vi "Test Combinations of Broken Wells.vi"(10 "broken streaks":u8[](array[numeric]), 11 "map":i8[](array[numeric])) -> (3 "possible combinations":u64)   [LabVIEW 2022 SP3]
uses:
  <vilib>/Utility/miscctls.llb/LVMapReplaceAction.ctl
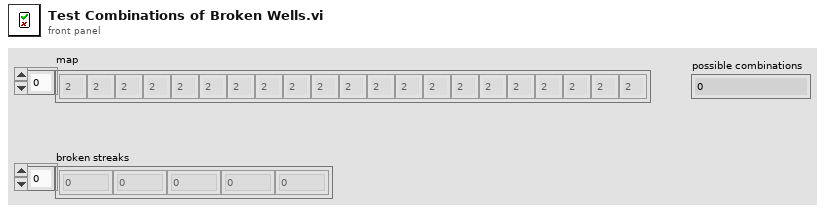
[diagram p1: front panel]
types:
  T1 = typedef "LVMapReplaceAction.ctl" = enum32{"Modify Entry only if found", "Add or Modify Entry", "Delete Entry"}
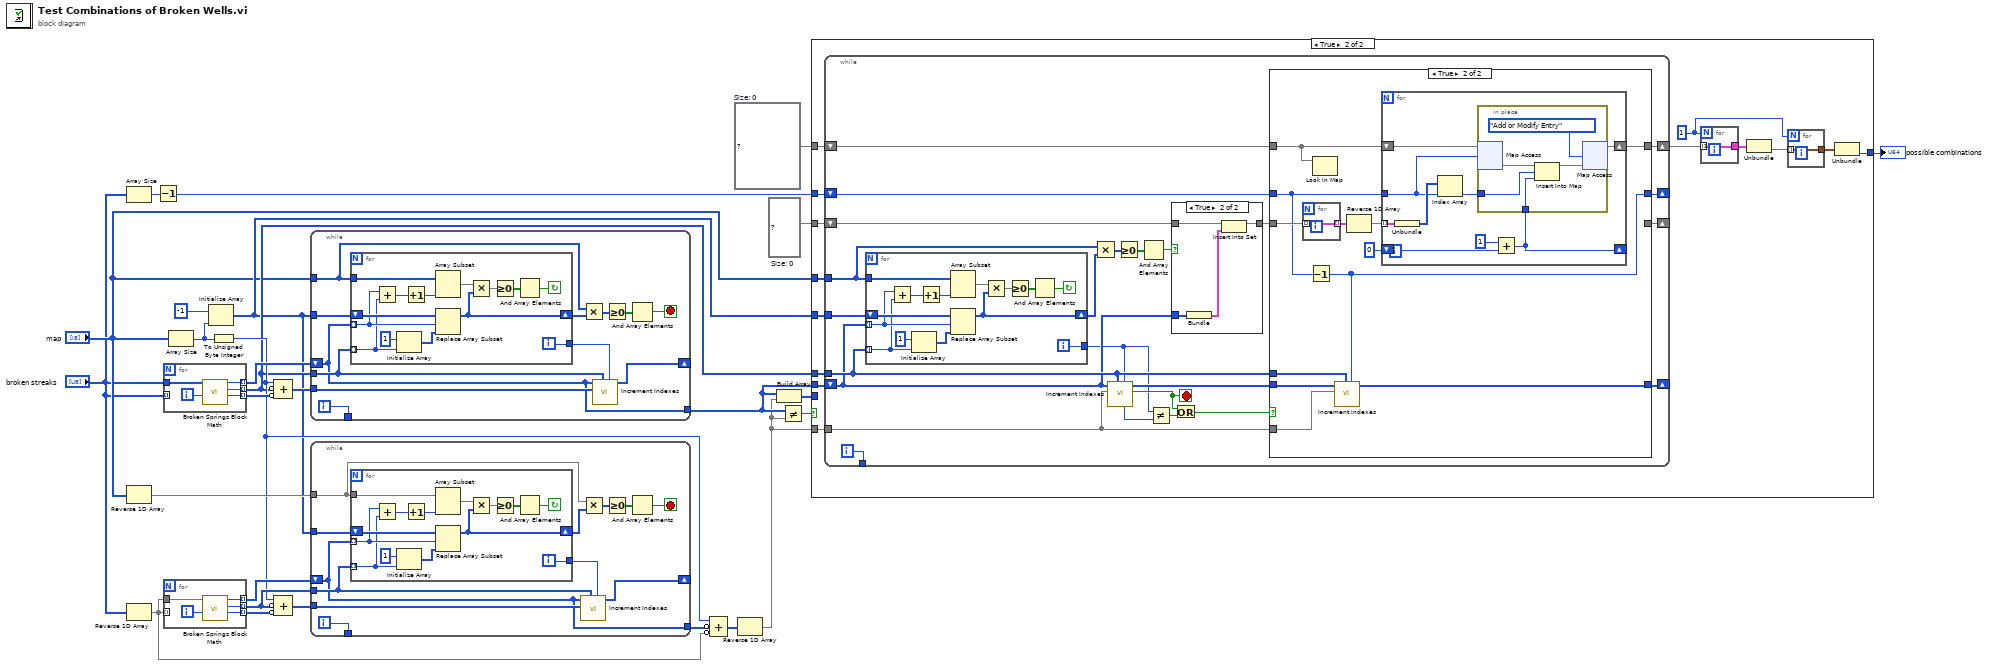
[diagram p0: block diagram]
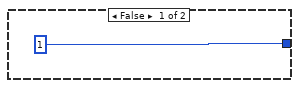
[diagram p2: hidden frame]
diagram:
  w5 = set{cluster{u8[]}} {}  # Size: 0
  w9 = map{i32, map{u8, u64}} {}  # Size: 0
  n1 = Array Size(array="broken streaks") -> (size(s)=w2:i32)
  n2 = Reverse 1D Array(array="map") -> (reversed array=w23:i8[])
  n3 = Reverse 1D Array(array="broken streaks") -> (reversed array=w17:u8[])
  n4 = Decrement(x=w2) -> (x-1=w1:i32)
  n5 = for {
    tunnel: "broken streaks" -> [w32]
    tunnel: "broken streaks" -> [_] mode=indexing
    tunnel: [w30] -> w26 mode=indexing
    tunnel: [w29] -> w11 mode=indexing
    tunnel: [w28] -> w27 mode=indexing
    i -> [w31]
    n6 = call "Broken Springs Block Math.vi"("index"=w31, "contiguous length of broken springs"=w32) -> ("right total"=w28:u8, "current index broken streak length"=w29:u8, "left total"=w30:u8)  [unwired: 7 in]
  }
  n7 = for {
    tunnel: w17 -> [w37]
    tunnel: w17 -> [_] mode=indexing
    tunnel: [w35] -> w21 mode=indexing
    tunnel: [w34] -> w20 mode=indexing
    tunnel: [w33] -> w22 mode=indexing
    i -> [w36]
    n8 = call "Broken Springs Block Math.vi"("index"=w36, "contiguous length of broken springs"=w37) -> ("right total"=w33:u8, "current index broken streak length"=w34:u8, "left total"=w35:u8)  [unwired: 7 in]
  }
  n9 = Array Size(array="map") -> (size(s)=w24:i32)
  n10 = Initialize Array(i8 -1 ("unsigned 8bit integer"), w24) -> (w10:i8[])
  n11 = To Unsigned Byte Integer(number=w24) -> (unsigned 8bit integer=w15:u8)
  n12 = Compound Arithmetic op=ADD(w15, invert w11, invert w27) -> (w14:u8[])
  n13 = Compound Arithmetic op=ADD(w15, invert w20, invert w22) -> (w19:u8[])
  n14 = while {
    tunnel: w10 -> [w49]
    tunnel: w11 -> [w46]
    shift-right: [w47] -> _
    shift-left: w26 -> [w43]
    tunnel: w14 -> [w48]
    tunnel: "map" -> [w38]
    tunnel: [w44] -> _
    tunnel: [w43] -> w13
    i -> [w44]
    stop <- w39 stop-if-true
    n15 = for {
      tunnel: w46 -> [w58] mode=indexing
      shift-right: [w55] -> w40
      shift-left: w49 -> [w63]
      tunnel: w43 -> [w59] mode=indexing
      tunnel: w38 -> [w60]
      tunnel: [w53] -> w45
      i -> [w53]
      stop <- w51 continue-if-true
      n16 = Add(x=w59, y=w58) -> (x+y=w57:u8)
      n17 = Initialize Array(i8 1 ("unsigned 8bit integer"), w58) -> (w62:i8[])
      n18 = Increment(x=w57) -> (x+1=w50:u8)
      n19 = Array Subset(array=w60, length=w50) -> (w56:i8[])  [unwired: 1 in]
      n20 = Replace Array Subset(array=w63, new element=w62, index=w59) -> (w55:i8[])
      n21 = Multiply(x=w56, y=w55) -> (x*y=w52:i8[])
      n22 = Greater Or Equal To 0?(x=w52) -> (x >= 0?=w54:bool[])
      n23 = And Array Elements(Boolean array=w54) -> (logical AND=w51:bool)
    }
    n24 = Multiply(x=w38, y=w40) -> (x*y=w41:i8[])
    n25 = call "Increment Indexes.vi"("group index to increment"=w45, "lengths"=w46, "max indexes"=w48, "previous indexes"=w43) -> ("next indexes"=w47:u8[])  [unwired: 5 in, 2 out]
    n26 = Greater Or Equal To 0?(x=w41) -> (x >= 0?=w42:bool[])
    n27 = And Array Elements(Boolean array=w42) -> (logical AND=w39:bool)
  }
  n28 = while {
    tunnel: w10 -> [w75]
    tunnel: w20 -> [w72]
    shift-right: [w73] -> _
    shift-left: w21 -> [w69]
    tunnel: w19 -> [w74]
    tunnel: w23 -> [w64]
    tunnel: [w70] -> _
    tunnel: [w69] -> w18
    i -> [w70]
    stop <- w66 stop-if-true
    n29 = for {
      tunnel: w72 -> [w84] mode=indexing
      shift-right: [w81] -> w65
      shift-left: w75 -> [w89]
      tunnel: w69 -> [w85] mode=indexing
      tunnel: w64 -> [w86]
      tunnel: [w79] -> w71
      i -> [w79]
      stop <- w77 continue-if-true
      n30 = Add(x=w85, y=w84) -> (x+y=w83:u8)
      n31 = Initialize Array(i8 1 ("unsigned 8bit integer"), w84) -> (w88:i8[])
      n32 = Increment(x=w83) -> (x+1=w76:u8)
      n33 = Array Subset(array=w86, length=w76) -> (w82:i8[])  [unwired: 1 in]
      n34 = Replace Array Subset(array=w89, new element=w88, index=w85) -> (w81:i8[])
      n35 = Multiply(x=w82, y=w81) -> (x*y=w78:i8[])
      n36 = Greater Or Equal To 0?(x=w78) -> (x >= 0?=w80:bool[])
      n37 = And Array Elements(Boolean array=w80) -> (logical AND=w77:bool)
    }
    n38 = call "Increment Indexes.vi"("group index to increment"=w71, "lengths"=w72, "max indexes"=w74, "previous indexes"=w69) -> ("next indexes"=w73:u8[])  [unwired: 5 in, 2 out]
    n39 = Multiply(x=w64, y=w65) -> (x*y=w68:i8[])
    n40 = Greater Or Equal To 0?(x=w68) -> (x >= 0?=w67:bool[])
    n41 = And Array Elements(Boolean array=w67) -> (logical AND=w66:bool)
  }
  n42 = Compound Arithmetic op=ADD(w15, invert w18, invert w17) -> (w16:u8[])
  n43 = Reverse 1D Array(array=w16) -> (reversed array=w12:u8[])
  n44 = Build Array(w13, w12) -> (w7:u8[][])
  n45 = Not Equal?(x=w13, y=w12) -> (x != y?=w8:bool)
  n46 = case shown="True" w8 {
    tunnel: "map" -> [_ w104]
    tunnel: w13 -> [_ w103]
    tunnel: w12 -> [_ w102]
    tunnel: w11 -> [_ w101]
    tunnel: w10 -> [_ w100]
    tunnel: w5 -> [_ w99]
    tunnel: w9 -> [_ w98]
    tunnel: w7 -> [_ _]
    tunnel: [u64 1 ("possible combinations") w97] -> w6
    tunnel: w1 -> [_ w91]
    frame False {
    }
    frame True {
      w92 = 1
      n47 = while {
        tunnel: w100 -> [w128]
        tunnel: w101 -> [w112]
        shift-right: [w114] -> _
        shift-left: w103 -> [w108]
        tunnel: w102 -> [w111]
        tunnel: w104 -> [w123]
        shift-right: [w116] -> _
        shift-left: w99 -> [w122]
        tunnel: [w127] -> _
        shift-right: [w109] -> w96
        shift-left: w98 -> [w110]
        shift-right: [w105] -> _
        shift-left: w91 -> [w106]
        i -> [w127]
        stop <- w118 stop-if-true
        n48 = for {
          tunnel: w112 -> [w137] mode=indexing
          shift-right: [w134] -> w124
          shift-left: w128 -> [w142]
          tunnel: w108 -> [w138] mode=indexing
          tunnel: w123 -> [w139]
          tunnel: [w132] -> w107
          i -> [w132]
          stop <- w130 continue-if-true
          n49 = Add(x=w138, y=w137) -> (x+y=w136:u8)
          n50 = Initialize Array(i8 1 ("unsigned 8bit integer"), w137) -> (w141:i8[])
          n51 = Increment(x=w136) -> (x+1=w129:u8)
          n52 = Array Subset(array=w139, length=w129) -> (w135:i8[])  [unwired: 1 in]
          n53 = Replace Array Subset(array=w142, new element=w141, index=w138) -> (w134:i8[])
          n54 = Multiply(x=w135, y=w134) -> (x*y=w131:i8[])
          n55 = Greater Or Equal To 0?(x=w131) -> (x >= 0?=w133:bool[])
          n56 = And Array Elements(Boolean array=w133) -> (logical AND=w130:bool)
        }
        n57 = Multiply(x=w123, y=w124) -> (x*y=w125:i8[])
        n58 = call "Increment Indexes.vi"("group index to increment"=w107, "lengths"=w112, "max indexes"=w111, "previous indexes"=w108) -> ("complete"=w118:bool, "next indexes"=w113:u8[], "actual index incremented"=w120:i32)  [unwired: 5 in]
        n59 = Greater Or Equal To 0?(x=w125) -> (x >= 0?=w126:bool[])
        n60 = And Array Elements(Boolean array=w126) -> (logical AND=w121:bool)
        n61 = Not Equal?(x=w107, y=w120) -> (x != y?=w119:bool)
        n62 = case shown="True" w121 {
          tunnel: w122 -> [w143 w147]
          tunnel: [w143 w146] -> w115
          tunnel: w108 -> [_ w145]
          frame False {
          }
          frame True {
            n63 = Bundle(w145) -> (w144:cluster{u8[]})  [unwired: 1 in]
            n64 = Insert Into Set(10:w144, 11:w147) -> (3:w146:set{cluster{u8[]}})  [unwired: 1 out]
          }
        }
        n65 = Or(x=w118, y=w119) -> (x .or. y?=w117:bool)
        n66 = case shown="True" w117 {
          tunnel: [w151 _] -> w116
          tunnel: w115 -> [w151 w159]
          tunnel: [w150 w162] -> w114
          tunnel: w113 -> [w150 w163]
          tunnel: w112 -> [_ w161]
          tunnel: w111 -> [_ w160]
          tunnel: w110 -> [w149 w152]
          tunnel: [w149 w156] -> w109
          tunnel: w106 -> [w148 w154]
          tunnel: [w148 w153] -> w105
          frame False {
          }
          frame True {
            n67 = for {
              tunnel: w159 -> [w178] mode=indexing
              tunnel: [w178] -> w158 mode=indexing
            }
            n68 = Decrement(x=w154) -> (x-1=w153:i32)
            n69 = Look In Map(map=w152) -> ()  [unwired: 2 in, 2 out]
            n70 = call "Increment Indexes.vi"("group index to increment"=w153, "lengths"=w161, "max indexes"=w160, "previous indexes"=w163) -> ("next indexes"=w162:u8[])  [unwired: 5 in, 2 out]
            n71 = Reverse 1D Array(array=w158) -> (reversed array=w157:cluster{u8[]}[])
            n72 = for {
              tunnel: w157 -> [w167] mode=indexing
              shift-right: [w169] -> w156
              shift-left: w152 -> [w170]
              tunnel: w154 -> [w165]
              shift-right: [w171] -> _
              shift-left: u64 0 -> [w172]
              n73 = Unbundle(w167) -> (w166:u8[])
              n74 = Index Array(array=w166, index=w165) -> (element=w164:u8)
              n75 = Add(x=u64 1, y=w172) -> (x+y=w171:u64)
              n76 = in-place {
                in-place-border: w171 -> [w177]
                in-place-border: w164 -> [w173]
                n77 = in-place-map #1(w170, w165) -> (w175:map{u8, u64})  [unwired: 1 in, 1 out]
                n78 = Insert Into Map(map in=w175, key=w173, value=w177) -> (map out=w174:map{u8, u64})  [unwired: 2 out]
                n79 = in-place-map #1(w174, LVMapReplaceAction."Add or Modify Entry" ("action")) -> (w169:map{i32, map{u8, u64}})  [unwired: 2 out]
              }
            }
          }
        }
      }
      n80 = for {
        N: w92 -> [_]
        tunnel: w96 -> [w179] mode=indexing
        tunnel: [w179] -> w95
      }
      n81 = Unbundle(w95) -> (w94:map{u8, u64})  [unwired: 1 out]
      n82 = for {
        N: w92 -> [_]
        tunnel: w94 -> [w180] mode=indexing
        tunnel: [w180] -> w93
      }
      n83 = Unbundle(w93) -> (w97:u64)  [unwired: 1 out]
    }
  }
  "possible combinations" <- w6
